vi "Write Row.vi"(8 "error in (no error)":errorcluster, 10 "Row":i32, 11 "2D Array in":refnum<class "2D Array.lvclass">) -> (0 "error out":errorcluster, 3 "2D Array out":refnum<class "2D Array.lvclass">)   [LabVIEW 2019, in "2D Array.lvclass"]
uses:
  2D Array.lvclass
  2D Array.lvclass/2D Array.ctl
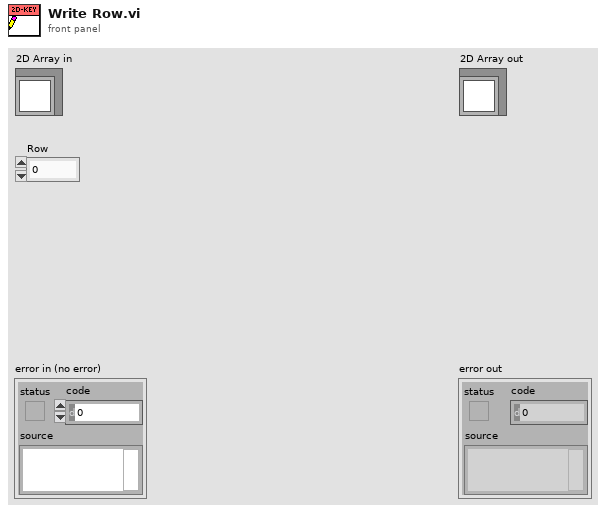
[diagram p1: front panel]
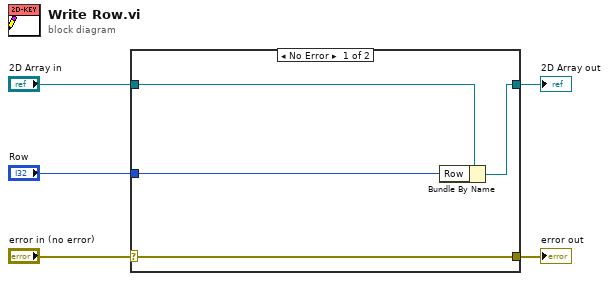
[diagram p0: block diagram]
diagram:
  n1 = case shown="No Error" "error in (no error)" {
    selector: "error in (no error)" -> [w9 w10]
    tunnel: [w9 w10] -> w4
    tunnel: [w7 w11] -> w2
    tunnel: "2D Array in" -> [w8 w11]
    tunnel: "Row" -> [w6 _]
    frame No Error {
      n2 = Bundle By Name(cluster=w8, "Row"=w6) -> (w7:refnum<class "2D Array.lvclass">)
    }
    frame Error {
    }
  }
  "error out" <- w4
  "2D Array out" <- w2
